vi "DMA.Scatter-Gather.Allocate Block Descriptor.vi"(8 "error in (no error)":errorcluster, 10 "block descriptor":T1 {"next descriptor ptr" format="%08x"; "data size" format="%08x"; "data ptr (upper)" format="%08x"; "data ptr (lower)" format="%08x"; "descriptor ptr (aligned)" format="%08x"; "descriptor size" format="%08x"; "descriptor ptr (VISA)" format="%08x"}, 11 "VISA Refnum in":refnum<visa-resource-name>) -> (0 "error out":errorcluster, 2 "allocated block descriptor":T2 {"Block Descriptor"."next descriptor ptr" format="%08x"; "Block Descriptor"."data size" format="%08x"; "Block Descriptor"."data ptr (upper)" format="%08x"; "Block Descriptor"."data ptr (lower)" format="%08x"; "Block Descriptor"."descriptor ptr (aligned)" format="%08x"; "Block Descriptor"."descriptor size" format="%08x"; "Block Descriptor"."descriptor ptr (VISA)" format="%08x"; "VISA size" format="%08x"; "VISA offset" format="%08x"}, 3 "VISA Refnum out":refnum<visa-resource-name>)   [LabVIEW 2016, in "GE 5565PIORC.lvclass"]
uses:
  GE 5565PIORC.lvclass
  Controls/DMA Block Descriptor (VISA).ctl
  Controls/DMA Block Descriptor.ctl
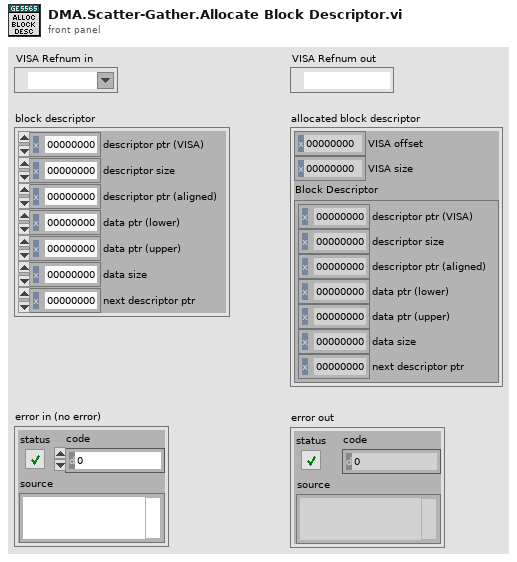
[diagram p1: front panel]
types:
  T1 = typedef "GE 5565PIORC.lvclass/DMA Block Descriptor.ctl" = cluster{"descriptor ptr (VISA)":u32, "descriptor size":u32, "descriptor ptr (aligned)":u32, "data ptr (lower)":u32, "data ptr (upper)":u32, "data size":u32, "next descriptor ptr":u32}
  T2 = typedef "GE 5565PIORC.lvclass/DMA Block Descriptor (VISA).ctl" = cluster{"VISA offset":u32, "VISA size":u32, "Block Descriptor":T1}
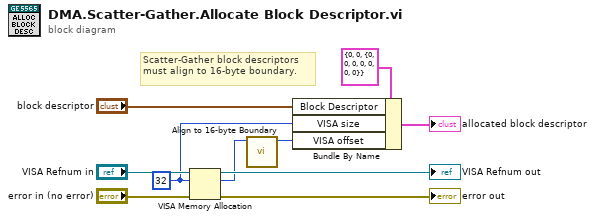
[diagram p0: block diagram]
diagram:
  w2 = u32 32 ("size")
  # "Scatter-Gather block descriptors must align to 16-byte boundary."
  n1 = VISA Memory Allocation(8:"error in (no error)", 10:w2, 11:"VISA Refnum in") -> (0:→"error out":errorcluster, 2:w1:u32, 3:→"VISA Refnum out":refnum<visa-resource-name>)
  n2 = call "Align to 16-byte Boundary.vi"("pointer"=w1) -> ("aligned pointer"=w6:u32)  [unwired: 10 in]
  n3 = Bundle By Name(cluster=T2 {"VISA offset"=0, "VISA size"=0, "Block Descriptor"={"descriptor ptr (VISA)"=0, "descriptor size"=0, "descriptor ptr (aligned)"=0, "data ptr (lower)"=0, "data ptr (upper)"=0, "data size"=0, "next descriptor ptr"=0}} ("Block Descriptor (VISA)"), "Block Descriptor"="block descriptor", "VISA size"=w2, "VISA offset"=w6) -> (→"allocated block descriptor":T2)
